vi "FGV Control Update.vi"(8 "error in":errorcluster, 10 "Function":T1, 11 "Enable Control Update":string[](array[string])) -> (0 "error out":errorcluster, 3 "Enable Control Update out":string[](array[string]))   [LabVIEW 2013]
uses:
  Device Drivers/shared/stop FGV control.ctl
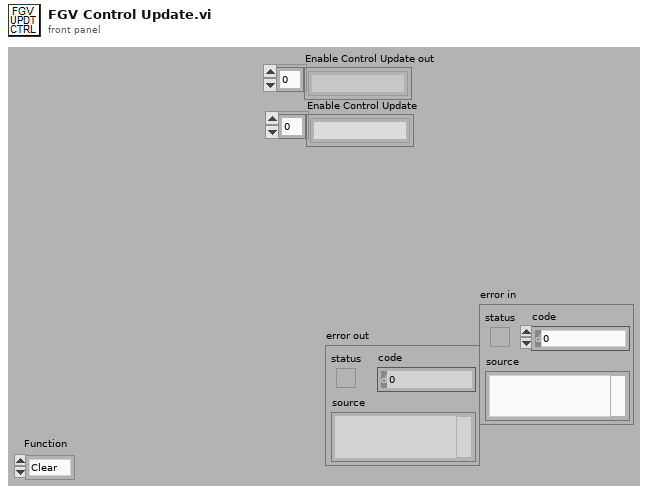
[diagram p1: front panel]
types:
  T1 = typedef "stop FGV control.ctl" = enum16{"Clear", "Write", "Read"}
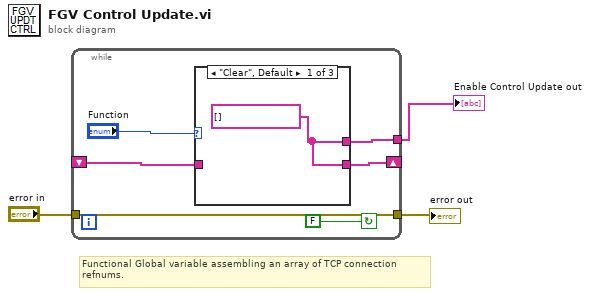
[diagram p0: block diagram]
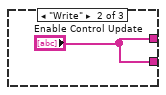
[diagram p2: hidden frame]
diagram:
  # "Functional Global variable assembling an array of TCP connection\nrefnums."
  n1 = while {
    shift-left: _ -> [w8]
    shift-right: [w9] -> _
    tunnel: [w5] -> w1
    tunnel: "error in" -> [w4]
    tunnel: [w4] -> w2
    stop <- FALSE continue-if-true
    n2 = case shown="\"Clear\", Default" "Function" {
      tunnel: [w10 "Enable Control Update" w12] -> w9
      tunnel: w8 -> [_ _ w12]
      tunnel: [w10 "Enable Control Update" w12] -> w5
      frame "Clear", Default {
        w10 = string[] []
      }
      frame "Write" {
      }
      frame "Read" {
      }
    }
  }
  "error out" <- w2
  "Enable Control Update out" <- w1
